vi "test starburst double.vi"() -> ()   [LabVIEW 2015]
uses:
  TCP client/TCP client.lvclass
  TCP/TCP server.lvclass
  connection/connection maintainer.lvclass
  communicator/communicator.lvclass
  <vilib>/ptbypt/NI_PtbyPt.lvlib
  message/communicator message.lvclass
  starburst/starburst.lvclass
  manager/queue manager.lvclass
  Queue server/Queue server.lvclass
  Queue Client/Queue client.lvclass
  communicator queue/enqueue variety.ctl
  communicator queue/identifying queue.lvclass
  communicator manager/communicator manager.lvlib
panel:
  out "ClienQ":refnum<class "identifying queue.lvclass">
  out "ClienQ 2":refnum<class "identifying queue.lvclass">
  out "ID 7":string
  out "data 7":variant
  out "ID 6":string
  out "data 6":variant
  out "ID 5":string
  out "data 5":variant
  out "Numeric 3":dbl
  out "ClienT 2":timestamp
  out "data 2":variant
  out "ID 2":string
  in  "remake c 2":bool
  in  "c2":cluster{"ID":string, "data":string}
  in  "C to S 2":bool
  out "Numeric 2":dbl
  out "data 3":variant
  out "ID 3":string
  out "data":variant
  out "ID":string
  out "Numeric":dbl
  in  "Boolean":bool
  in  "remake c":bool
  in  "s":cluster{"ID":string, "data":string}
  in  "c1":cluster{"ID":string, "data":string}
  in  "S to C":bool
  in  "C to S":bool
  in  "exits":bool
  out "ClienT":timestamp
  out "servT":timestamp
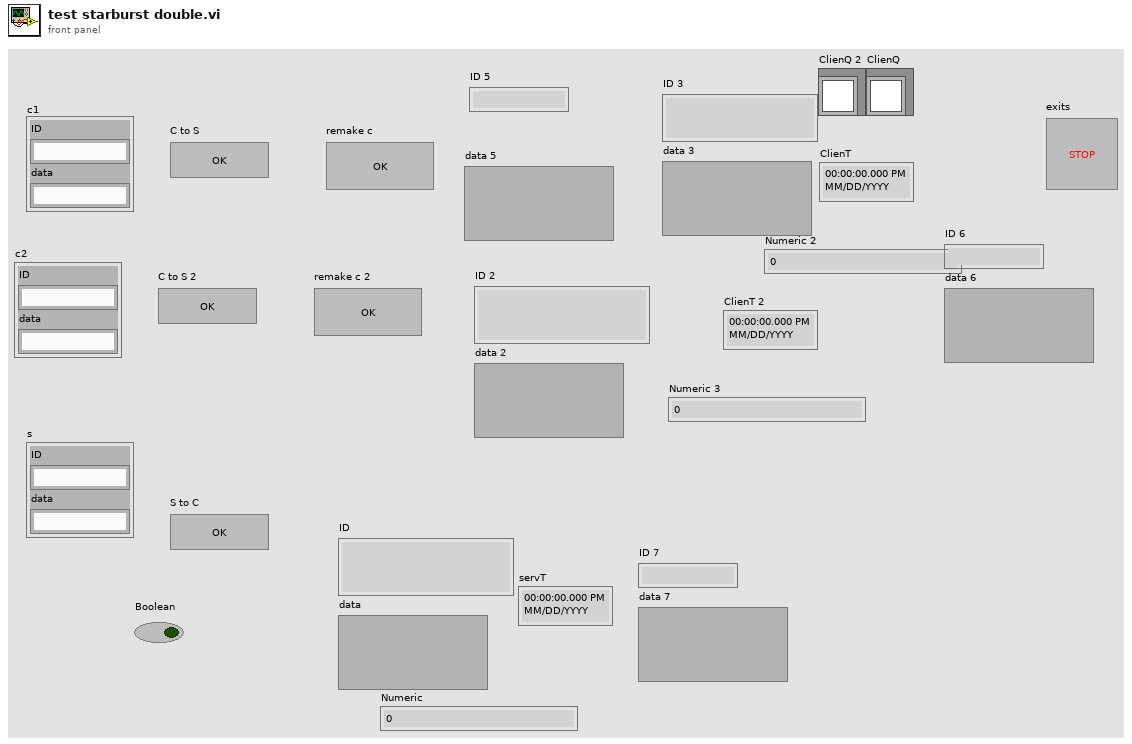
[diagram p1: front panel]
types:
  T1 = typedef "identifying queue.lvclass/enqueue variety.ctl" = enum16{"normal", "lossy", "priority"}
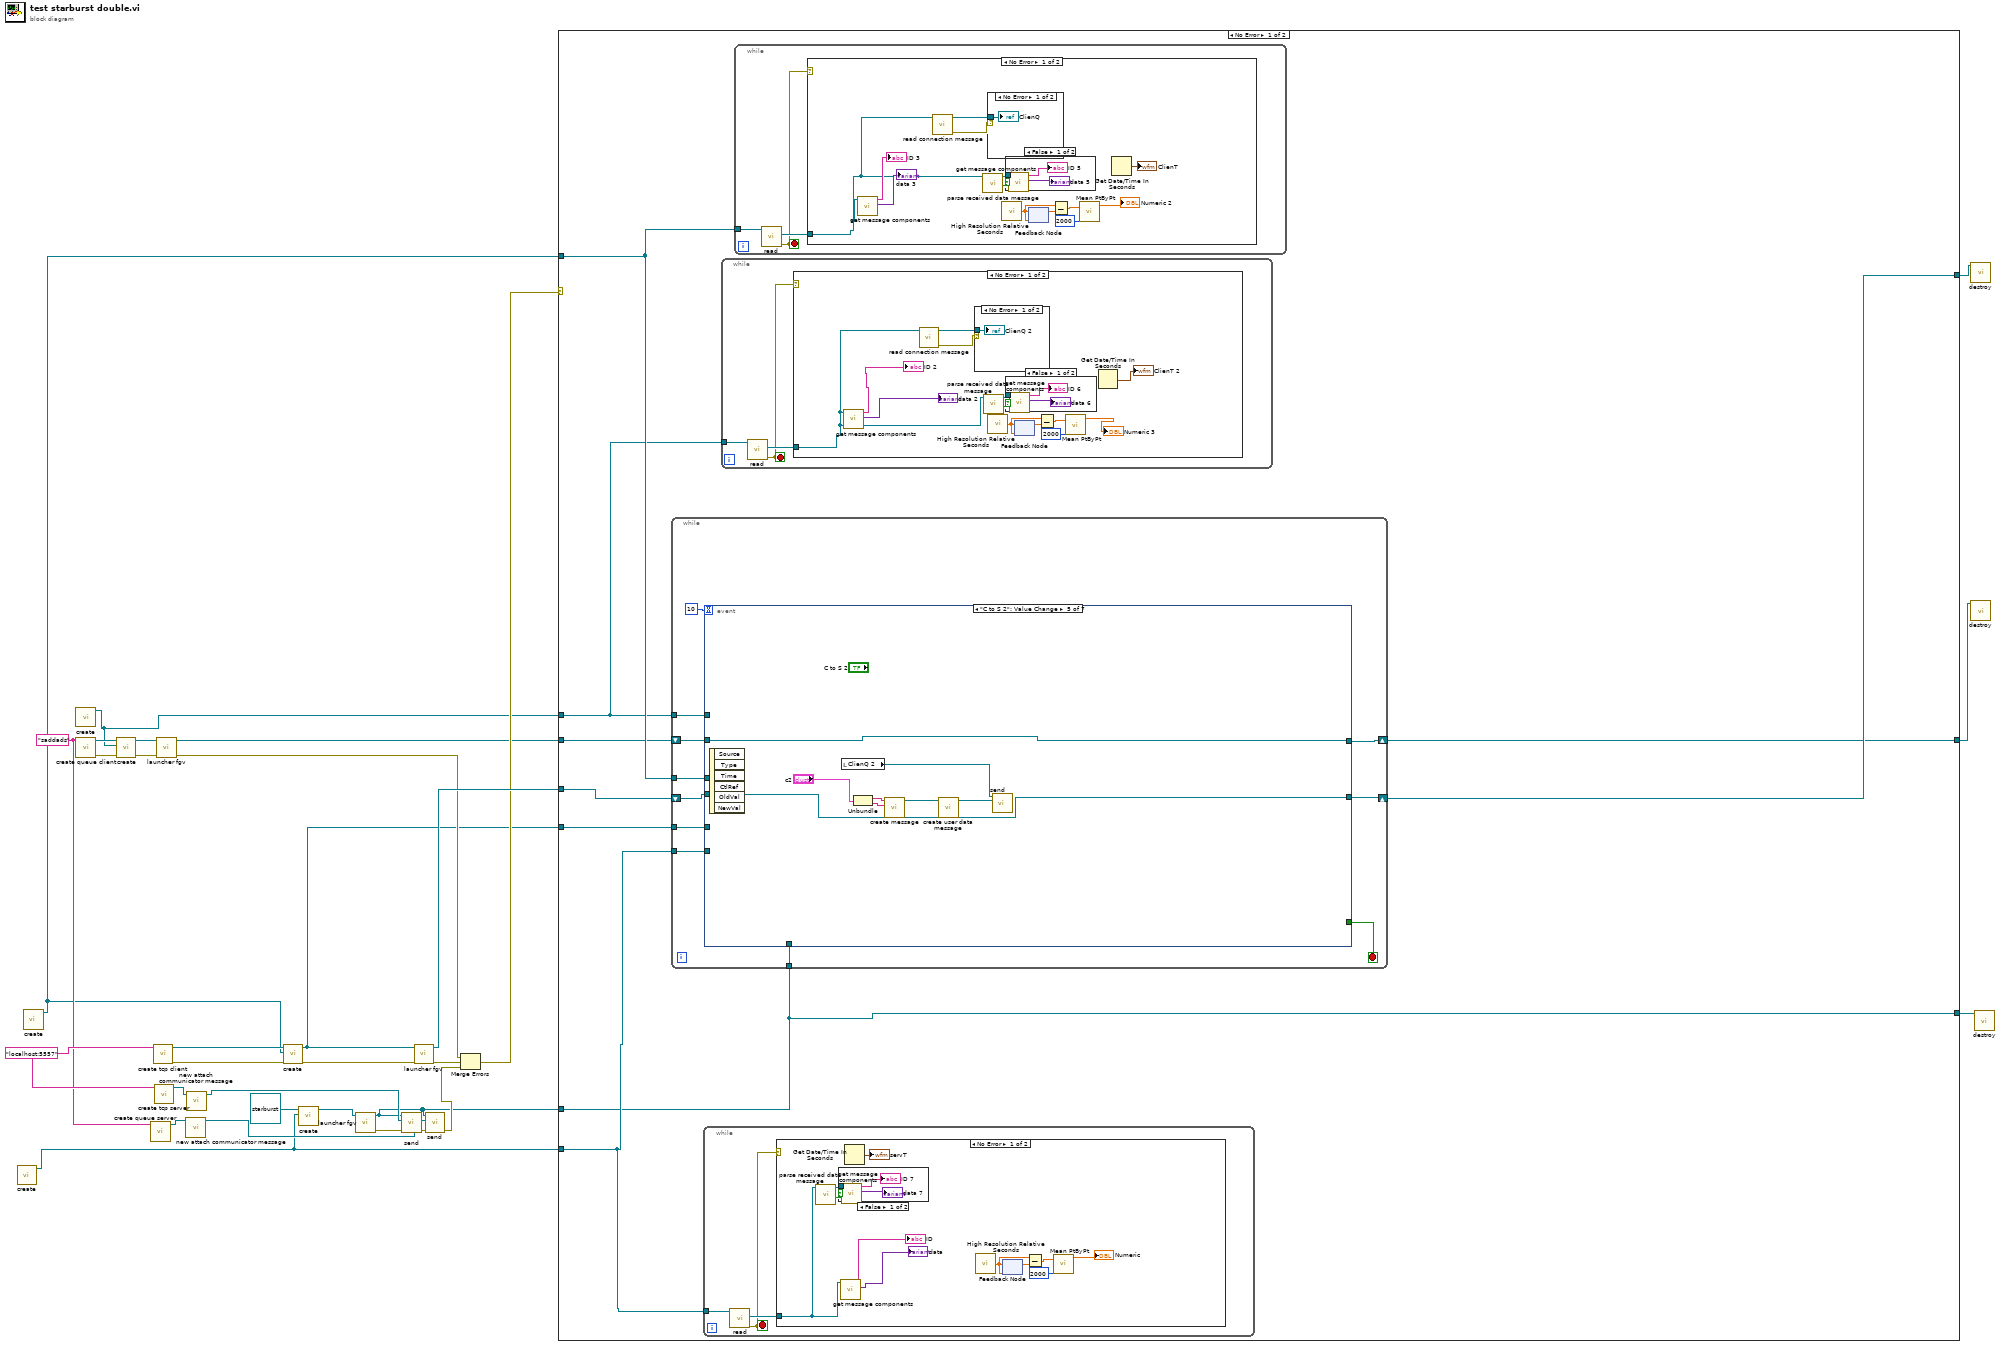
[diagram p0: block diagram]
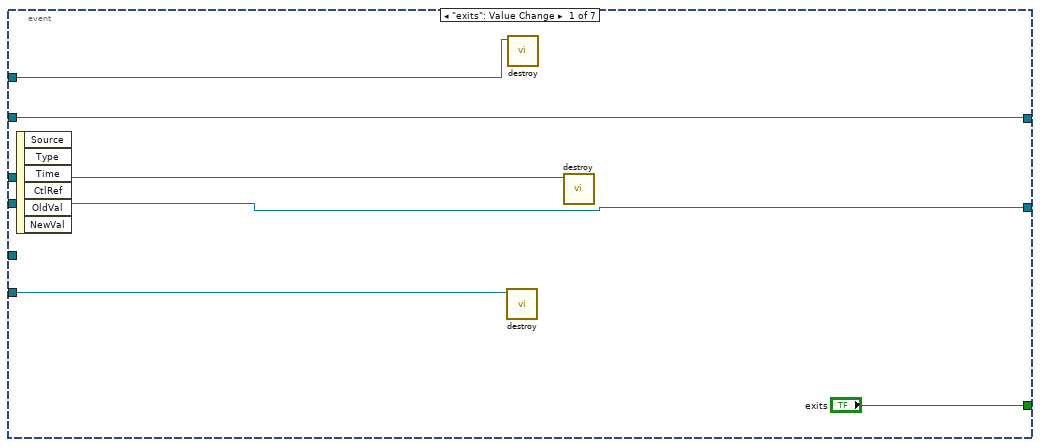
[diagram p5: hidden frame]
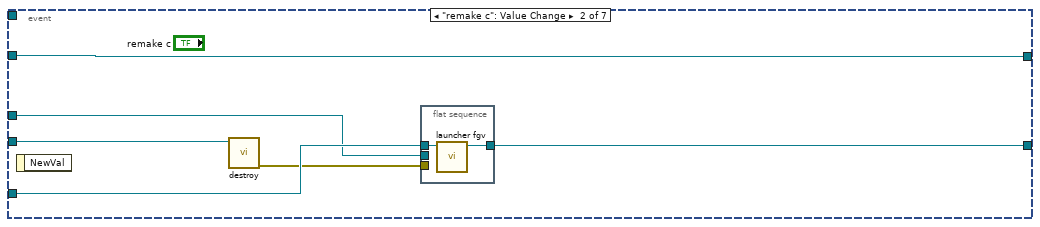
[diagram p6: hidden frame]
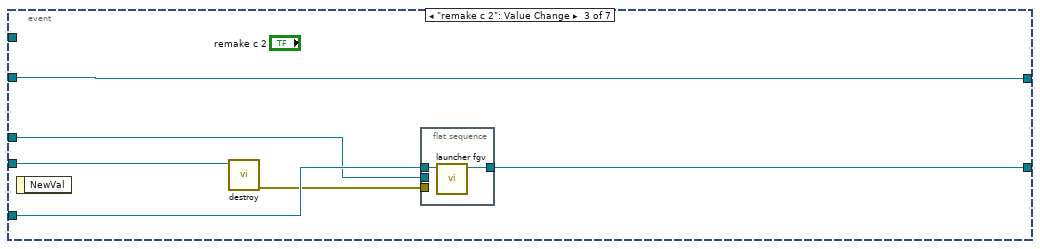
[diagram p7: hidden frame]
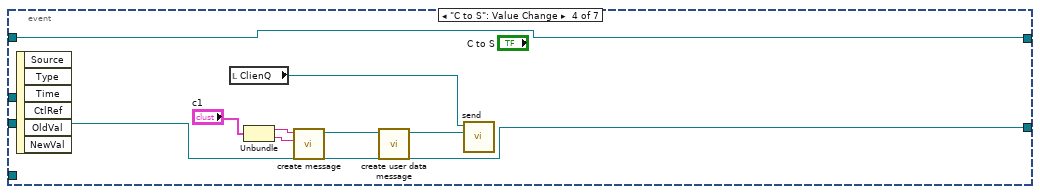
[diagram p8: hidden frame]
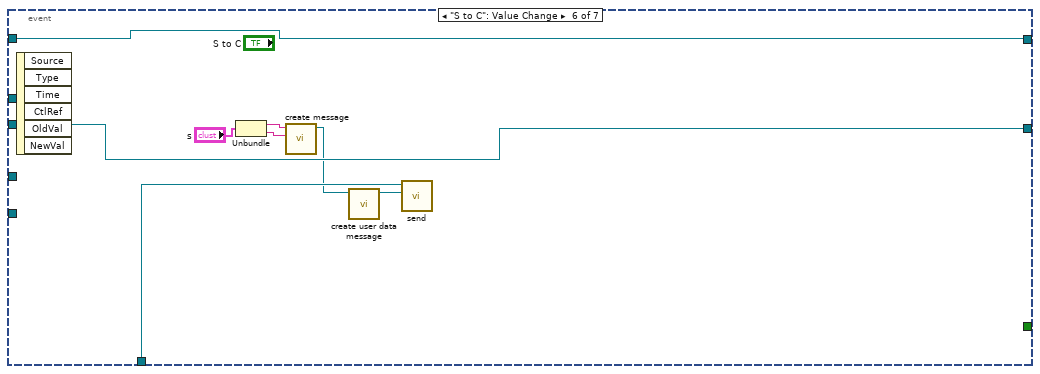
[diagram p9: hidden frame]
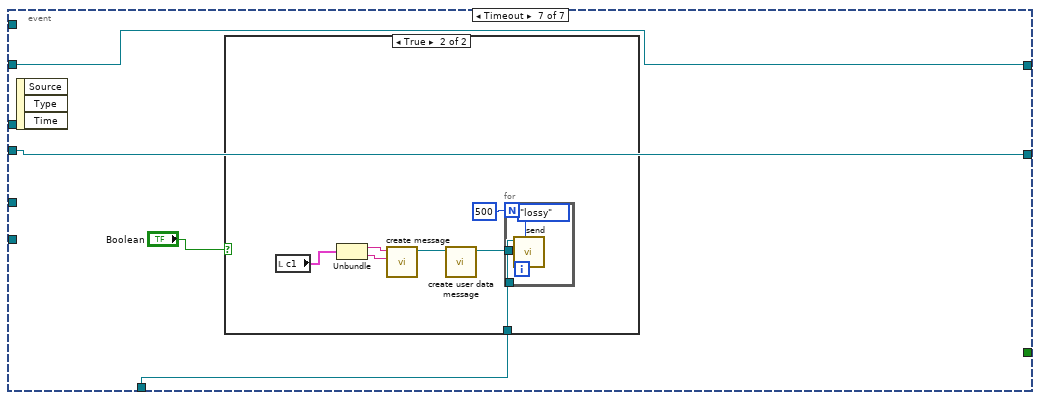
[diagram p10: hidden frame]
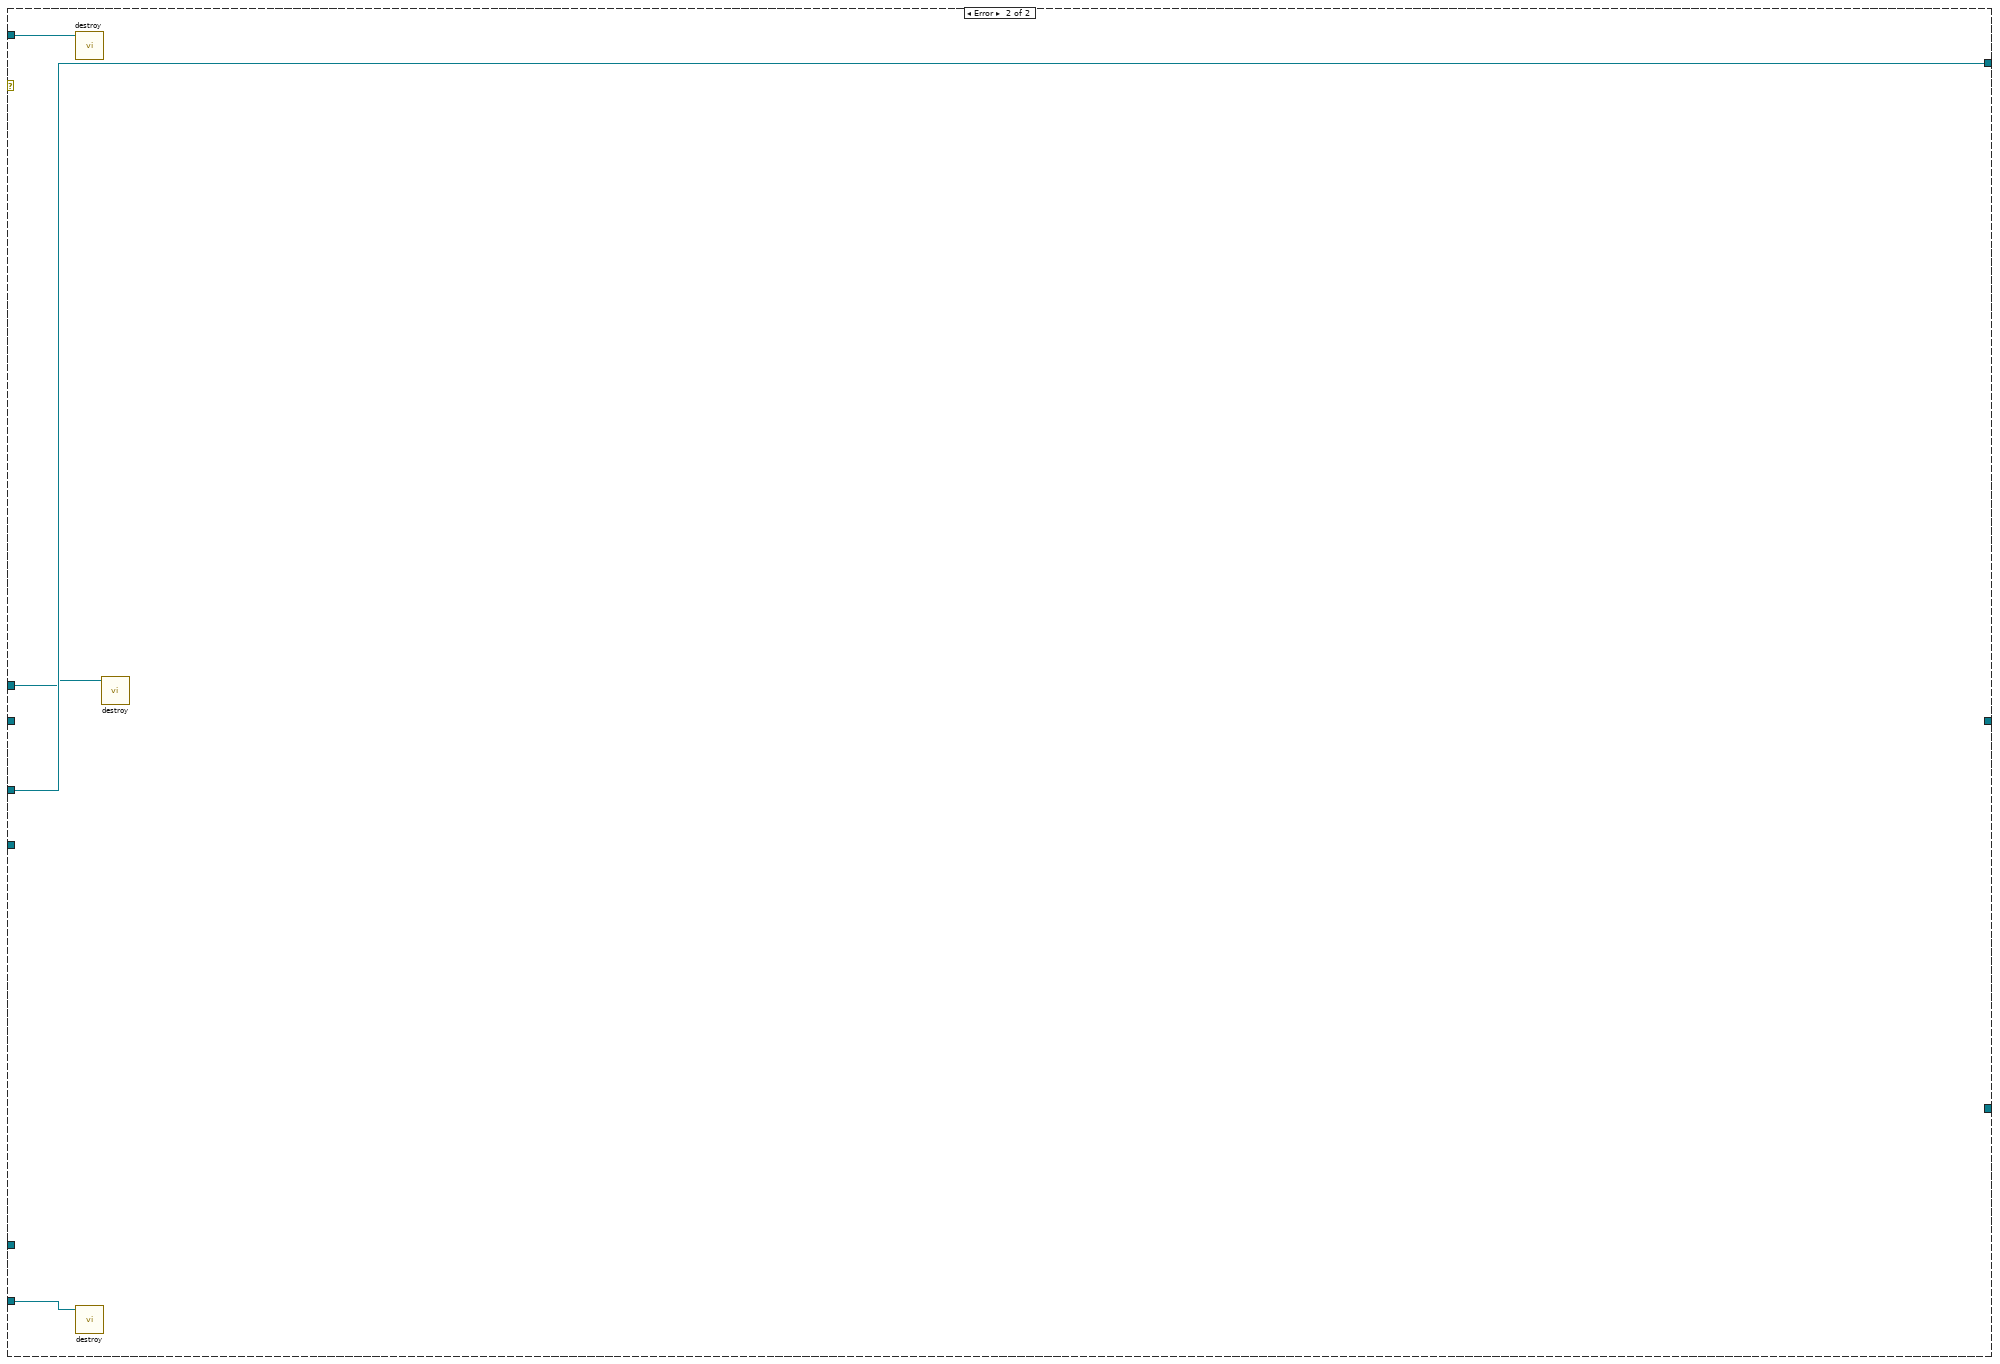
[diagram p17: hidden frame]
diagram:
  w11 = "saddads" ("connection string")
  w27 = "localhost:5557" ("connection string")
  n1 = call "create.vi"() -> ("message connection out"=w5:refnum<class "identifying queue.lvclass">)  [unwired: 10 in, 1 out]
  n2 = call "create.vi"() -> ("message connection out"=w7:refnum<class "identifying queue.lvclass">)  [unwired: 10 in, 1 out]
  n3 = call "create.vi"() -> ("message connection out"=w1:refnum<class "identifying queue.lvclass">)  [unwired: 10 in, 1 out]
  n4 = call "create queue client.vi"("conn string"=w11) -> ("error out"=w15:errorcluster, "TCP client out"=w3:refnum<class "Queue client.lvclass">)  [unwired: 9 in]
  n5 = call "create.vi"("error in"=w15, "parent"=w1, "uninitialized communicator"=w3) -> ("error out"=w4:errorcluster, "communicator out"=w2:refnum<class "Queue client.lvclass">)  [unwired: 7 in]
  n6 = call "create queue server.vi"("conn string"=w11) -> ("TCP server out"=w19:refnum<class "Queue server.lvclass">)  [unwired: 9 in, 1 out]
  n7 = call "create tcp client.vi"("conn string"=w27) -> ("error out"=w30:errorcluster, "TCP client out"=w9:refnum<class "TCP client.lvclass">)  [unwired: 9 in]
  n8 = call "create tcp server.vi"("conn string"=w27) -> ("TCP server out"=w23:refnum<class "TCP server.lvclass">)  [unwired: 9 in, 1 out]
  n9 = call "launcher fgv.vi"("error in"=w4, "communicator in"=w2) -> ("error out"=w14:errorcluster, "initialized communicator"=w13:refnum<class "communicator.lvclass">)  [unwired: 8 in]
  n10 = call "new attach communicator message.vi"("comm"=w19) -> ("message"=w16:refnum<class "communicator message.lvclass">)  [unwired: 10 in]
  n11 = call "new attach communicator message.vi"("comm"=w23) -> ("message"=w21:refnum<class "communicator message.lvclass">)  [unwired: 10 in]
  n12 = call "create.vi"("error in"=w30, "parent"=w7, "uninitialized communicator"=w9) -> ("error out"=w10:errorcluster, "communicator out"=w8:refnum<class "TCP client.lvclass">)  [unwired: 7 in]
  n13 = call "create.vi"("parent"=w5, "uninitialized communicator"=refnum<class "starburst.lvclass"> refnum ("starburst")) -> ("communicator out"=w6:refnum<class "starburst.lvclass">)  [unwired: 8 in, 1 out]
  n14 = call "launcher fgv.vi"("communicator in"=w6) -> ("error out"=w24:errorcluster, "initialized communicator"=w17:refnum<class "communicator.lvclass">)  [unwired: 9 in]
  n15 = call "send.vi"("error in"=w24, "element"=w21, "communicator in"=w17) -> ("error out"=w22:errorcluster)  [unwired: 8 in]
  n16 = call "launcher fgv.vi"("error in"=w10, "communicator in"=w8) -> ("error out"=w28:errorcluster, "initialized communicator"=w29:refnum<class "communicator.lvclass">)  [unwired: 8 in]
  n17 = call "send.vi"("error in"=w22, "element"=w16, "communicator in"=w17) -> ("error out"=w18:errorcluster)  [unwired: 8 in]
  n18 = Merge Errors(w14, w28, w18) -> (w26:errorcluster)
  n19 = case shown="No Error" w26 {
    tunnel: [w36 w171] -> w31
    tunnel: w7 -> [w39 w172]
    tunnel: w29 -> [w38 w171]
    tunnel: w5 -> [w40 w170]
    tunnel: w8 -> [w37 _]
    tunnel: w17 -> [w35 _]
    tunnel: [w35 _] -> w20
    tunnel: w13 -> [w34 _]
    tunnel: w1 -> [w33 w169]
    tunnel: [w32 _] -> w12
    frame No Error {
      n20 = while {
        tunnel: w40 -> [w70]
        tunnel: w39 -> [w69]
        tunnel: w37 -> [w67]
        shift-right: [w66] -> w36
        shift-left: w38 -> [w68]
        tunnel: w35 -> [w64]
        shift-right: [w61] -> w32
        shift-left: w34 -> [w63]
        tunnel: w33 -> [w62]
        stop <- w71 stop-if-true
        n21 = event shown="[4] \"C to S 2\": Value Change" {
          selector: _ -> [_ _ _ _ _ _ _]
          dyn-events: _ -> [_ _ _ _ _ _ _]
          timeout: 10 -> [_ _ _ _ _ _ _]
          tunnel: ["exits" _ _ _ _ _ _] -> w71
          tunnel: w70 -> [w76 _ _ _ _ _ _]
          tunnel: w69 -> [w75 w80 w88 _ _ _ _]
          tunnel: w68 -> [w74 w83 w91 w99 w107 w117 w121]
          tunnel: w67 -> [_ w82 w90 _ _ _ _]
          tunnel: [w74 w79 w87 w99 w107 w117 w121] -> w66
          tunnel: w64 -> [_ _ _ _ _ w113 w119]
          tunnel: w63 -> [w73 w78 w86 w95 w104 w111 w118]
          tunnel: w62 -> [w72 _ _ _ _ _ _]
          tunnel: [w73 w78 w86 w95 w104 w111 w118] -> w61
          event "exits": Value Change {
            n22 = event-data() -> ()  [unwired: 1 in, 6 out]
            n23 = call "destroy.vi"("message connection in"=w76) -> ()  [unwired: 10 in, 1 out]
            n24 = call "destroy.vi"("message connection in"=w72) -> ()  [unwired: 10 in, 1 out]
            n25 = call "destroy.vi"("message connection in"=w75) -> ()  [unwired: 10 in, 1 out]
          }
          event "remake c": Value Change {
            n26 = event-data() -> ()  [unwired: 1 in, 1 out]
            n27 = call-dynamic "destroy.vi"("communicator in"=w83) -> ("error out"=w81:errorcluster)  [unwired: 10 in]
            n28 = flat-sequence {
              tunnel: w82 -> [w85]
              tunnel: w81 -> [_]
              tunnel: w80 -> [_]
              tunnel: [w84] -> w79
              frame #0 {
                n29 = call "launcher fgv.vi"("communicator in"=w85) -> ("initialized communicator"=w84:refnum<class "communicator.lvclass">)  [unwired: 9 in, 1 out]
              }
            }
          }
          event "remake c 2": Value Change {
            n30 = event-data() -> ()  [unwired: 1 in, 1 out]
            n31 = call-dynamic "destroy.vi"("communicator in"=w91) -> ("error out"=w89:errorcluster)  [unwired: 10 in]
            n32 = flat-sequence {
              tunnel: w90 -> [w93]
              tunnel: w89 -> [_]
              tunnel: w88 -> [_]
              tunnel: [w92] -> w87
              frame #0 {
                n33 = call "launcher fgv.vi"("communicator in"=w93) -> ("initialized communicator"=w92:refnum<class "communicator.lvclass">)  [unwired: 9 in, 1 out]
              }
            }
          }
          event "C to S": Value Change {
            n34 = event-data() -> ()  [unwired: 1 in, 6 out]
            n35 = local read "ClienQ"() -> (w101:refnum<class "identifying queue.lvclass">)
            n36 = Unbundle("c1") -> ("ID"=w98:string, "data"=w97:string)
            n37 = call "create message.vi"("data"=w97, "ID"=w98) -> ("message"=w100:refnum<class "communicator message.lvclass">)  [unwired: 9 in]
            n38 = call "create user data message.vi"("data"=w100) -> ("message"=w94:refnum<class "communicator message.lvclass">)  [unwired: 10 in]
            n39 = call "send.vi"("message"=w94, "message connection in"=w101) -> ()  [unwired: 8 in, 2 out]
          }
          event "C to S 2": Value Change {
            n40 = event-data() -> ()  [unwired: 1 in, 6 out]
            n41 = local read "ClienQ 2"() -> (w109:refnum<class "identifying queue.lvclass">)
            n42 = Unbundle("c2") -> ("ID"=w106:string, "data"=w105:string)
            n43 = call "create message.vi"("data"=w105, "ID"=w106) -> ("message"=w108:refnum<class "communicator message.lvclass">)  [unwired: 9 in]
            n44 = call "create user data message.vi"("data"=w108) -> ("message"=w102:refnum<class "communicator message.lvclass">)  [unwired: 10 in]
            n45 = call "send.vi"("message"=w102, "message connection in"=w109) -> ()  [unwired: 8 in, 2 out]
          }
          event "S to C": Value Change {
            n46 = event-data() -> ()  [unwired: 1 in, 6 out]
            n47 = Unbundle("s") -> ("ID"=w116:string, "data"=w115:string)
            n48 = call "create message.vi"("data"=w115, "ID"=w116) -> ("message"=w112:refnum<class "communicator message.lvclass">)  [unwired: 9 in]
            n49 = call "create user data message.vi"("data"=w112) -> ("message"=w110:refnum<class "communicator message.lvclass">)  [unwired: 10 in]
            n50 = call "send.vi"("element"=w110, "communicator in"=w113) -> ()  [unwired: 9 in, 1 out]
          }
          event Timeout {
            n51 = event-data() -> ()  [unwired: 1 in, 3 out]
            n52 = case shown="True" "Boolean" {
              tunnel: w119 -> [_ w124]
              frame False {
              }
              frame True {
                n53 = local read "c1"() -> (w126:cluster{"ID":string, "data":string})
                n54 = Unbundle(w126) -> ("ID"=w128:string, "data"=w127:string)
                n55 = call "create message.vi"("data"=w127, "ID"=w128) -> ("message"=w125:refnum<class "communicator message.lvclass">)  [unwired: 9 in]
                n56 = call "create user data message.vi"("data"=w125) -> ("message"=w122:refnum<class "communicator message.lvclass">)  [unwired: 10 in]
                n57 = for {
                  N: 500 -> [_]
                  tunnel: w122 -> [w131]
                  tunnel: w124 -> [w130]
                  n58 = call "send.vi"("enqueue setting"=enqueue_variety."lossy", "element"=w131, "communicator in"=w130) -> ()  [unwired: 8 in, 1 out]
                }
              }
            }
          }
        }
      }
      n59 = while {
        tunnel: w40 -> [w134]
        stop <- w132 stop-if-true
        n60 = call "read.vi"("identifying queue in"=w134) -> ("error out"=w132:errorcluster, "message"=w133:refnum<class "communicator message.lvclass">)  [unwired: 8 in, 1 out]
        n61 = case shown="No Error" w132 {
          tunnel: w133 -> [w135 _]
          frame No Error {
            n62 = call "parse received data message.vi"("message"=w135) -> ("invalid?"=w136:bool, "data"=w137:refnum<class "communicator message.lvclass">)  [unwired: 9 in]
            n63 = case shown="False" w136 {
              tunnel: w137 -> [w148 _]
              frame False {
                n64 = call "get message components.vi"("message"=w148) -> ("data"=→"data 7":variant, "ID"=→"ID 7":string)  [unwired: 9 in]
              }
              frame True {
              }
            }
            n65 = call "get message components.vi"("message"=w135) -> ("data"=→"data":variant, "ID"=→"ID":string)  [unwired: 9 in]
            n66 = Get Date/Time In Seconds() -> (seconds since 1Jan1904=→"servT":timestamp)
            n67 = call <vilib>:"High Resolution Relative Seconds.vi"() -> ("relative seconds"=w143:dbl)
            n68 = feedback-in #1(w143) -> ()
            n69 = feedback #1(w143) -> (w144:dbl)
            n70 = Subtract(x=w143, y=w144) -> (x-y=w142:dbl)
            n71 = call <vilib>:"Mean PtByPt.vi"("x"=w142, "sample length"=2000) -> ("mean"=→"Numeric":dbl)  [unwired: 2 in, 1 out]
          }
          frame Error {
          }
        }
      }
      n72 = while {
        tunnel: w33 -> [w43]
        stop <- w41 stop-if-true
        n73 = call "read.vi"("identifying queue in"=w43) -> ("error out"=w41:errorcluster, "message"=w42:refnum<class "communicator message.lvclass">)  [unwired: 8 in, 1 out]
        n74 = case shown="No Error" w41 {
          tunnel: w42 -> [w44 _]
          frame No Error {
            n75 = call "get message components.vi"("message"=w44) -> ("data"=→"data 2":variant, "ID"=→"ID 2":string)  [unwired: 9 in]
            n76 = call "read connection message.vi"("communicator message in"=w44) -> ("error out"=w55:errorcluster, "queue"=w56:refnum<class "identifying queue.lvclass">)  [unwired: 9 in]
            n77 = case shown="No Error" w55 {
              tunnel: w56 -> [w60 _]
              frame No Error {
                "ClienQ 2" <- w60
              }
              frame Error {
              }
            }
            n78 = call "parse received data message.vi"("message"=w44) -> ("invalid?"=w45:bool, "data"=w46:refnum<class "communicator message.lvclass">)  [unwired: 9 in]
            n79 = call <vilib>:"High Resolution Relative Seconds.vi"() -> ("relative seconds"=w52:dbl)
            n80 = case shown="False" w45 {
              tunnel: w46 -> [w59 _]
              frame False {
                n81 = call "get message components.vi"("message"=w59) -> ("data"=→"data 6":variant, "ID"=→"ID 6":string)  [unwired: 9 in]
              }
              frame True {
              }
            }
            n82 = feedback #2(w52) -> (w51:dbl)
            n83 = feedback-in #2(w52) -> ()
            n84 = Subtract(x=w52, y=w51) -> (x-y=w53:dbl)
            n85 = call <vilib>:"Mean PtByPt.vi"("x"=w53, "sample length"=2000) -> ("mean"=→"Numeric 3":dbl)  [unwired: 2 in, 1 out]
            n86 = Get Date/Time In Seconds() -> (seconds since 1Jan1904=→"ClienT 2":timestamp)
          }
          frame Error {
          }
        }
      }
      n87 = while {
        tunnel: w39 -> [w151]
        stop <- w149 stop-if-true
        n88 = call "read.vi"("identifying queue in"=w151) -> ("error out"=w149:errorcluster, "message"=w150:refnum<class "communicator message.lvclass">)  [unwired: 8 in, 1 out]
        n89 = case shown="No Error" w149 {
          tunnel: w150 -> [w152 _]
          frame No Error {
            n90 = call "get message components.vi"("message"=w152) -> ("data"=→"data 3":variant, "ID"=→"ID 3":string)  [unwired: 9 in]
            n91 = call "read connection message.vi"("communicator message in"=w152) -> ("error out"=w163:errorcluster, "queue"=w164:refnum<class "identifying queue.lvclass">)  [unwired: 9 in]
            n92 = call "parse received data message.vi"("message"=w152) -> ("invalid?"=w154:bool, "data"=w153:refnum<class "communicator message.lvclass">)  [unwired: 9 in]
            n93 = case shown="No Error" w163 {
              tunnel: w164 -> [w168 _]
              frame No Error {
                "ClienQ" <- w168
              }
              frame Error {
              }
            }
            n94 = call <vilib>:"High Resolution Relative Seconds.vi"() -> ("relative seconds"=w156:dbl)
            n95 = case shown="False" w154 {
              tunnel: w153 -> [w167 _]
              frame False {
                n96 = call "get message components.vi"("message"=w167) -> ("data"=→"data 5":variant, "ID"=→"ID 5":string)  [unwired: 9 in]
              }
              frame True {
              }
            }
            n97 = feedback #3(w156) -> (w155:dbl)
            n98 = feedback-in #3(w156) -> ()
            n99 = Subtract(x=w156, y=w155) -> (x-y=w157:dbl)
            n100 = call <vilib>:"Mean PtByPt.vi"("x"=w157, "sample length"=2000) -> ("mean"=→"Numeric 2":dbl)  [unwired: 2 in, 1 out]
            n101 = Get Date/Time In Seconds() -> (seconds since 1Jan1904=→"ClienT":timestamp)
          }
          frame Error {
          }
        }
      }
    }
    frame Error {
      n102 = call "destroy.vi"("message connection in"=w172) -> ()  [unwired: 10 in, 1 out]
      n103 = call "destroy.vi"("message connection in"=w170) -> ()  [unwired: 10 in, 1 out]
      n104 = call "destroy.vi"("message connection in"=w169) -> ()  [unwired: 10 in, 1 out]
    }
  }
  n105 = call-dynamic "destroy.vi"("communicator in"=w31) -> ()  [unwired: 10 in, 1 out]
  n106 = call-dynamic "destroy.vi"("communicator in"=w12) -> ()  [unwired: 10 in, 1 out]
  n107 = call-dynamic "destroy.vi"("communicator in"=w20) -> ()  [unwired: 10 in, 1 out]
